vi "Generate Linear Accel Segment.vi"(4 "Stoopid Overlap distance":dbl min=0.0, 6 "Index":i32, 7 "Initial Acceleration":dbl format="%#_13g", 8 "Velocities":dbl[](array[numeric]), 9 "Linear Info":T2, 10 "Stoopid V":dbl=20.0, 11 "Speeds in":T1={"maxV (fps)"=20.0, "Accel Limit (fps^2)"=20.0, "Initial V (fps)"=0.0, "Sample Period (s)"=0.02, "Jerk Limit (fps^3)"=0.0, "Distances"=[]}) -> (0 "Valid":bool, 1 "Final Position":cluster{dbl, dbl, dbl}, 2 "Trajectory Segment":T3, 3 "Speeds out":T1={"maxV (fps)"=20.0, "Accel Limit (fps^2)"=20.0, "Initial V (fps)"=0.0, "Sample Period (s)"=0.02, "Jerk Limit (fps^3)"=0.0, "Distances"=[]}, 5 "Final Acceleration":dbl)   [LabVIEW 2019]
uses:
  Speeds.ctl
panel:
  out "Waveform Graph":dbl[][](graph)
  out "XY Graph":cluster{dbl, dbl}[](graph)
  out "Segment Time (s)":dbl
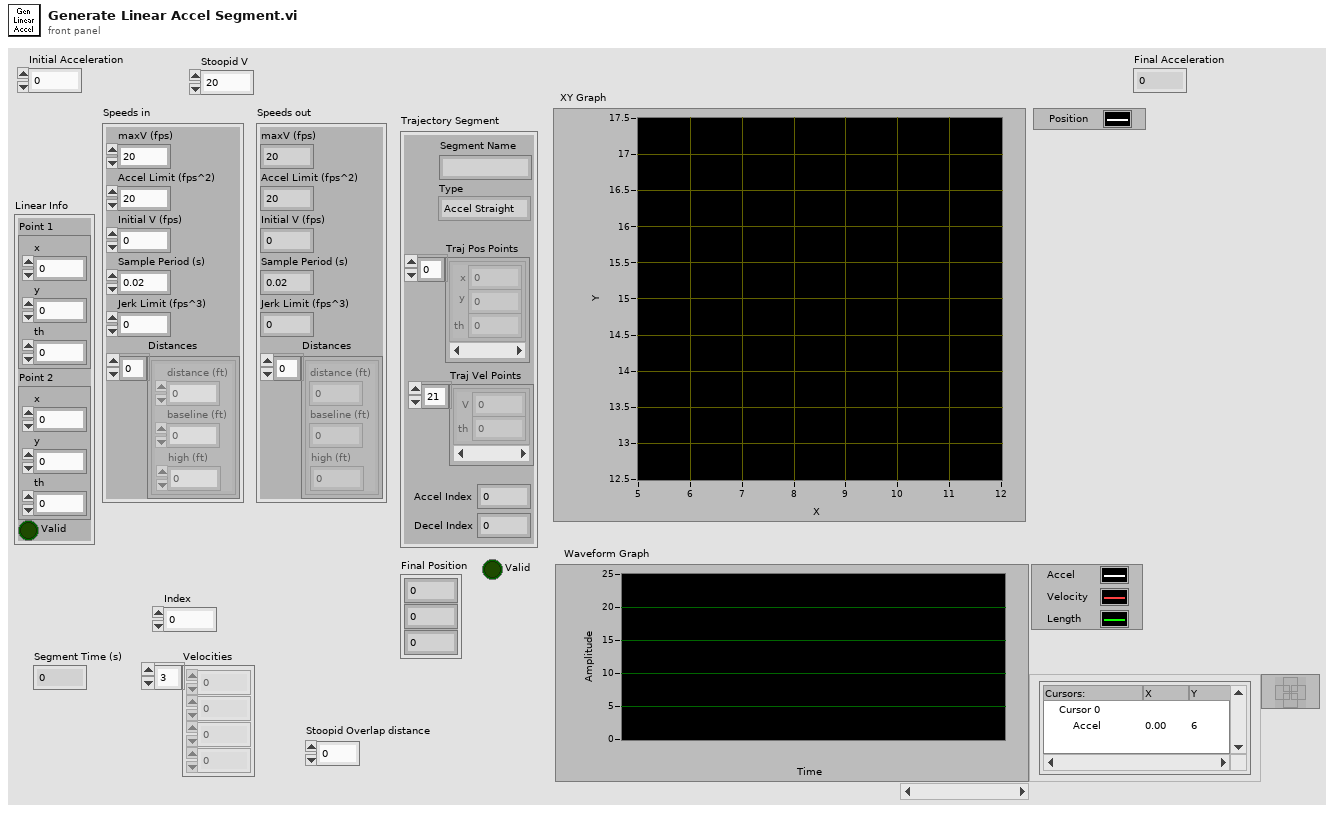
[diagram p1: front panel]
types:
  T1 = typedef "Speeds.ctl" = cluster{"maxV (fps)":dbl, "Accel Limit (fps^2)":dbl, "Initial V (fps)":dbl, "Sample Period (s)":dbl, "Jerk Limit (fps^3)":dbl, "Distances":cluster{"distance (ft)":dbl, "baseline (ft)":dbl, "high (ft)":dbl}[]}
  T2 = cluster{"Point 1":cluster{"x":dbl, "y":dbl, "th":dbl}, "Point 2":cluster{"x":dbl, "y":dbl, "th":dbl}, "Valid":bool}
  T3 = cluster{"Segment Name":string, "Type":enum16{"Accel Straight", "Const Straight", "Blend", "Circle"}, "Traj Pos Points":cluster{"x":dbl, "y":dbl, "th":dbl}[], "Traj Vel Points":cluster{"V":dbl, "th":dbl}[], "Accel Index":i32, "Decel Index":i32}
  T4 = enum16{"Accel Straight", "Const Straight", "Blend", "Circle"}
  T5 = cluster{"Accel Limit (fps^2)":dbl, "Jerk Limit (fps^3)":dbl}
  T6 = cluster{"distance (ft)":dbl, "dist baseline jerk":dbl, "dist of high Jerk":dbl}[]
  T7 = cluster{"Initial Acceleration":dbl, "Initial V (fps)":dbl}
  T8 = cluster{string, "Type":enum16{"Accel Straight", "Const Straight", "Blend", "Circle"}, cluster{dbl, dbl, dbl}[], cluster{"velocity":dbl, dbl}[], "Accel Index":i32, "Decel Index":i32}
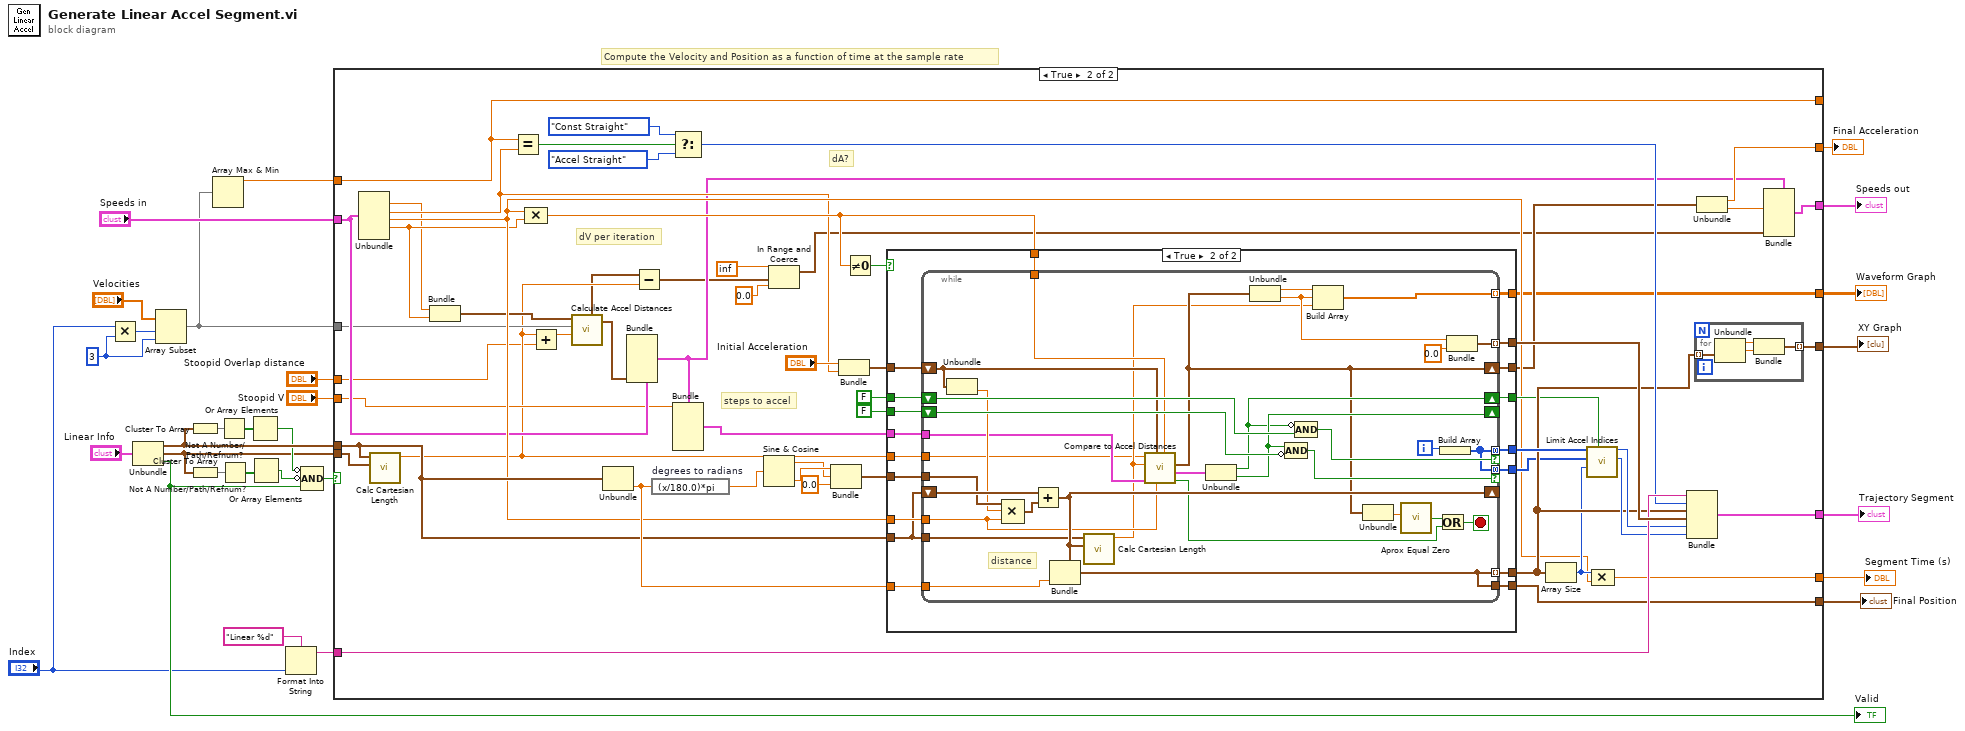
[diagram p0: block diagram]
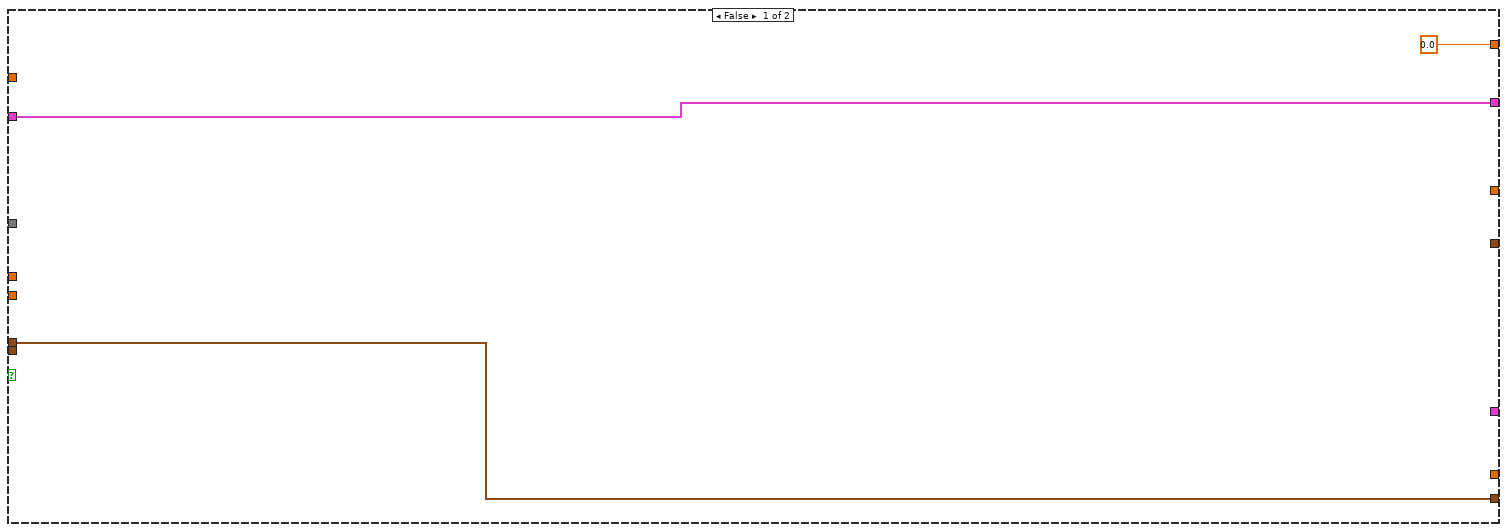
[diagram p2: hidden frame]
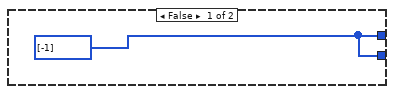
[diagram p3: hidden frame]
diagram:
  w6 = 3
  # "Compute the Velocity and Position as a function of time at the sample rate"
  n1 = Multiply(x="Index", y=w6) -> (x*y=w8:i32)
  n2 = Unbundle("Linear Info") -> ("Point 1"=w18:cluster{"x":dbl, "y":dbl, "th":dbl}, "Point 2"=w13:cluster{"x":dbl, "y":dbl, "th":dbl}, "Valid"=w19:bool)
  "Valid" <- w19
  n3 = Array Subset(array="Velocities", index=w8, length=w6) -> (w4:dbl[])
  n4 = Cluster To Array(cluster=w18) -> (array=w17:dbl[])
  n5 = Cluster To Array(cluster=w13) -> (array=w14:dbl[])
  n6 = Array Max & Min(array=w4) -> (max value=w3:dbl)  [unwired: 3 out]
  n7 = Not A Number/Path/Refnum?(number/path/refnum=w17) -> (NaN/Path/Refnum?=w16:bool[])
  n8 = Not A Number/Path/Refnum?(number/path/refnum=w14) -> (NaN/Path/Refnum?=w12:bool[])
  n9 = Or Array Elements(Boolean array=w16) -> (logical OR=w15:bool)
  n10 = Or Array Elements(Boolean array=w12) -> (logical OR=w11:bool)
  n11 = Format Into String(format string="Linear %d", "Index") -> (resulting string=w21:string)  [unwired: 2 in, 1 out]
  n12 = Compound Arithmetic op=AND(invert w15, invert w11, w19) -> (w20:bool)
  n13 = case shown="True" w20 {
    tunnel: [_ w88] -> w29
    tunnel: w21 -> [_ w82]
    tunnel: [_ w78] -> w28
    tunnel: [w31 w77] -> w27
    tunnel: [_ w74] -> w26
    tunnel: "Speeds in" -> [w32 w47]
    tunnel: [w32 w73] -> w24
    tunnel: w18 -> [w31 w68]
    tunnel: w13 -> [_ w71]
    tunnel: [_ w52] -> w10
    tunnel: [0.0 w51] -> w9
    tunnel: w4 -> [_ w46]
    tunnel: w3 -> [_ w45]
    tunnel: "Stoopid V" -> [_ w42]
    tunnel: [_ w45] -> _
    tunnel: "Stoopid Overlap distance" -> [_ w36]
    frame False {
    }
    frame True {
      # "dA?"
      # "steps to accel"
      # "dV per iteration"
      n14 = Unbundle(w47) -> ("Accel Limit (fps^2)"=w49:dbl, "Initial V (fps)"=w56:dbl, "Sample Period (s)"=w58:dbl, "Jerk Limit (fps^3)"=w50:dbl)  [unwired: 2 out]
      n15 = call "Calc Cartesian Length.vi"("Point 2"=w71, "Point 1"=w68) -> ("Length (f)"=w41:dbl)  [unwired: 8 in, 1 out]
      n16 = Bundle("Accel Limit (fps^2)"=w49, "Jerk Limit (fps^3)"=w50) -> (w48:T5)  [unwired: 1 in]
      n17 = Equal?(x=w45, y=w56) -> (x = y?=w72:bool)
      n18 = Compound Arithmetic op=MULTIPLY(w58, w50) -> (w70:dbl)
      n19 = Add(x=w41, y=w36) -> (x+y=w35:dbl)
      n20 = call "Calculate Accel Distances.vi"("Length (f)"=w35, "Velocities"=w46, "Limits"=w48) -> ("Distances"=w34:T6, "Const V Dist"=w33:T6)  [unwired: 7 in]
      n21 = Unbundle(w68) -> ("th"=w76:dbl)  [unwired: 2 out]
      n22 = Bundle(cluster=w47, "Distances"=w34) -> (w44:T1)  [unwired: 5 in]
      n23 = Subtract(x=w33, y=w41) -> (x-y=w38:T6)
      n24 = expression code="(x/180.0)*pi" "degrees to radians"(w76) -> (w75:dbl)
      n25 = Select(t=T4."Const Straight" ("Type"), s=w72, f=T4."Accel Straight" ("Type")) -> (s? t:f=w79:T4)
      n26 = Bundle(cluster=w44, "maxV (fps)"=w42) -> (w43:T1)  [unwired: 5 in]
      n27 = Sine & Cosine(0:w75) -> (1:w83:dbl, 2:w84:dbl)
      n28 = In Range and Coerce(upper limit=inf, x=w38, lower limit=0.0) -> (coerced(x)=w37:T6)  [unwired: 1 out]
      n29 = Bundle(w84, w83, 0.0) -> (w86:cluster{dbl, dbl, dbl})  [unwired: 1 in]
      n30 = Bundle("Initial Acceleration"="Initial Acceleration", "Initial V (fps)"=w56) -> (w55:T7)  [unwired: 1 in]
      n31 = Not Equal To 0?(x=w70) -> (x != 0?=w69:bool)
      n32 = case shown="True" w69 {
        tunnel: [_ w111] -> w87
        tunnel: w86 -> [_ w110]
        tunnel: [_ w109] -> w77
        tunnel: w76 -> [_ w108]
        tunnel: [_ w107] -> w62
        tunnel: [_ w106] -> w54
        tunnel: w70 -> [_ w105]
        tunnel: w58 -> [_ w104]
        tunnel: w68 -> [_ w103]
        tunnel: FALSE -> [_ w102]
        tunnel: [w93 w101] -> w65
        tunnel: w43 -> [_ w100]
        tunnel: FALSE -> [_ w99]
        tunnel: [w93 w98] -> w61
        tunnel: [_ w97] -> w59
        tunnel: w55 -> [_ w96]
        tunnel: [_ w95] -> w52
        tunnel: w41 -> [_ w94]
        frame False {
          w93 = i32[] [-1]
        }
        frame True {
          n33 = while {
            tunnel: [w136] -> w107 mode=indexing
            tunnel: w105 -> [w123]
            shift-right: [w116] -> w106
            shift-left: w96 -> [w126]
            tunnel: [w142] -> w111 mode=indexing
            tunnel: w104 -> [w120]
            tunnel: w110 -> [w140]
            tunnel: w108 -> [w143]
            tunnel: [w136] -> w109
            shift-right: [w138] -> _
            shift-left: w103 -> [w141]
            tunnel: w103 -> [w137]
            shift-right: [w122] -> w97
            shift-left: w102 -> [w134]
            tunnel: [w131] -> w101 mode=concatenating if=w133
            tunnel: w100 -> [w119]
            shift-right: [w125] -> _
            shift-left: w99 -> [w132]
            tunnel: [w131] -> w98 mode=concatenating if=w130
            tunnel: [w121] -> w95 mode=indexing
            tunnel: w94 -> [w114]
            i -> [w135]
            stop <- w129 stop-if-true
            # "distance"
            n34 = Unbundle(w126) -> ("Initial V (fps)"=w127:dbl)  [unwired: 1 out]
            n35 = Compound Arithmetic op=MULTIPLY(w140, w127, w120) -> (w139:cluster{dbl, dbl, dbl})
            n36 = Add(x=w141, y=w139) -> (x+y=w138:cluster{dbl, dbl, dbl})
            n37 = Bundle(cluster=w138, w143) -> (w136:cluster{dbl, dbl, dbl})  [unwired: 2 in]
            n38 = call "Calc Cartesian Length.vi"("Point 2"=w138, "Point 1"=w137) -> ("Length (f)"=w115:dbl)  [unwired: 8 in, 1 out]
            n39 = call "Compare to Accel Distances.vi"("dA"=w123, "Sample Period (s)"=w120, "Values"=w126, "Speeds in"=w119, "Current  Length"=w115, "Total Segment Length"=w114) -> ("End Loop"=w112:bool, "Ends"=w113:cluster{"Accel End":bool, "Decel End":bool}, "Values out"=w116:cluster{"accel":dbl, "velocity":dbl})  [unwired: 2 in, 1 out]
            n40 = Unbundle(w113) -> ("Accel End"=w122:bool, "Decel End"=w125:bool)
            n41 = Unbundle(w116) -> ("accel"=w117:dbl, "velocity"=w118:dbl)
            n42 = Compound Arithmetic op=AND(w125, invert w132) -> (w130:bool)
            n43 = Compound Arithmetic op=AND(invert w122, w134) -> (w133:bool)
            n44 = Build Array(w117, w118, w115) -> (w121:dbl[])
            n45 = Unbundle(w116) -> ("velocity"=w124:dbl)  [unwired: 1 out]
            n46 = call "Aprox Equal Zero.vi"("maxV (fps)"=w124) -> ("Boolean"=w128:bool)  [unwired: 10 in]
            n47 = Or(x=w128, y=w112) -> (x .or. y?=w129:bool)
            n48 = Build Array(w135) -> (w131:i32[])
            n49 = Bundle("velocity"=w118, 0.0) -> (w142:cluster{"velocity":dbl, dbl})  [unwired: 1 in]
          }
        }
      }
      n50 = Array Size(array=w62) -> (size(s)=w60:i32)
      n51 = call "Limit Accel Indices.vi"("Last Accel"=w59, "Size"=w60, "Decel"=w61, "Accel"=w65) -> ("Decel Index"=w64:i32, "Accel Index"=w66:i32)  [unwired: 6 in]
      n52 = Compound Arithmetic op=MULTIPLY(w60, w58) -> (w78:dbl)
      n53 = Bundle(w82, "Type"=w79, w62, w87, "Accel Index"=w66, "Decel Index"=w64) -> (w88:T8)  [unwired: 1 in]
      n54 = for {
        tunnel: w62 -> [w92] mode=indexing
        tunnel: [w89] -> w74 mode=indexing
        n55 = Unbundle(w92) -> (w91:dbl, w90:dbl)  [unwired: 1 out]
        n56 = Bundle(w91, w90) -> (w89:cluster{dbl, dbl})  [unwired: 1 in]
      }
      n57 = Unbundle(w54) -> ("Initial Acceleration"=w51:dbl, "Initial V (fps)"=w53:dbl)
      n58 = Bundle(cluster=w44, "Initial V (fps)"=w53, "Distances"=w37) -> (w73:T1)  [unwired: 4 in]
    }
  }
  "Trajectory Segment" <- w29
  "Segment Time (s)" <- w28
  "Final Position" <- w27
  "XY Graph" <- w26
  "Speeds out" <- w24
  "Waveform Graph" <- w10
  "Final Acceleration" <- w9
